vi "Get Data.vi"(8 "error in":errorcluster, 11 "PAS HF UI in":refnum<class "PAS HF UI.lvclass">) -> (0 "error out":errorcluster, 1 "Stop?":bool, 2 "Data":refnum<class "Data.lvclass">, 3 "PAS HF UI out":refnum<class "PAS HF UI.lvclass">)   [LabVIEW 2012, in "PAS HF UI.lvclass"]
uses:
  PAS HF UI.lvclass
  Reusable/GUI/GUI.lvclass
  Reusable/Data/Data.lvclass
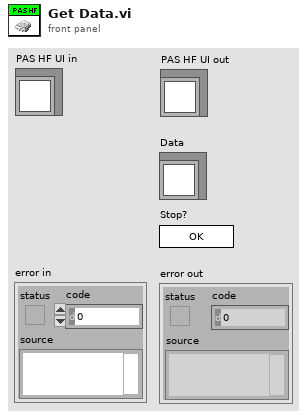
[diagram p1: front panel]
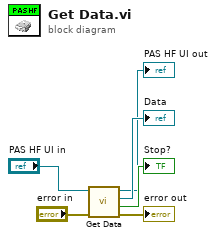
[diagram p0: block diagram]
diagram:
  n1 = call-parent "Get Data.vi"("error in"="error in", "PAS UI In"="PAS HF UI in") -> ("error out"=→"error out":errorcluster, "Stop?"=→"Stop?":bool, "Data"=→"Data":refnum<class "Data.lvclass">, "PAS UI Out"=→"PAS HF UI out":refnum<class "PAS UI.lvclass">)  [unwired: 6 in]
